vi "example_01_timescaledb.vi"() -> ()   [LabVIEW 2015, in "lv-timescaledb.lvlib"]
uses:
  lv-timescaledb.lvlib
  public/_controls/hypertable_options.ctl
  public/_controls/chunk.ctl
  public/_controls/time_type.ctl
  <vilib>/addons/database/Connection.llb/Conn ObjectReference.ctl
  <vilib>/addons/database/Connection.llb/DB Tools Open Connec (String).vi
  <vilib>/addons/database/NI_Database_API.lvlib
panel:
  out "connected?":bool
  in  "driver":string="PostgreSQL ANSI"
  in  "disconnect":bool
  in  "connect":bool
  in  "server":string="localhost"
  in  "password":string="timescaledb"
  in  "username":string="timescaledb"
  in  "chunk_name":string
  in  "hyper_table_name":string
  in  "tab_control":T1(tab)
  in  "hypertable_options":T2={"time_column"="time", "chunk_time_interval"=0.0} {"chunk_time_interval" format="%<%H:%M:%S>t"}
  in  "create_hypertable":bool
  in  "set_chunk_time_interval":bool
  in  "chunk_time_interval":dbl=86400.0 format="%<%H:%M:%S>t"
  in  "enable_compression":bool
  in  "segment_column":string="time"
  in  "disable_compression":bool
  in  "show_hyper_tables":bool
  out "hyper_tables":string[](array[string])
  in  "show_chunks":bool
  out "chunks_available []":T3[](array[typedef]) {"start" format="%^<%H:%M:%S%3u %m/%d/%y>T"; "end" format="%^<%H:%M:%S%3u %m/%d/%y>T"}
  out "decompressed_chunk":string
  out "compressed_chunk":string
  in  "decompress_chunk":bool
  in  "compress_chunk":bool
  in  "time_type":T4=enum."interval"
  in  "drop_chunks":bool
  out "chunks_dropped []":string[](array[string])
  in  "older_than_timestamp":dbl format="%^<%H:%M:%S%3u %m/%d/%y>T"
  in  "older_than_interval":dbl format="%<%H:%M:%S%4u>t"
  in  "newer_than_timestamp":dbl format="%^<%H:%M:%S%3u %m/%d/%y>T"
  in  "newer_than_interval":dbl format="%<%H:%M:%S%4u>t"
  in  "timezone":string
  in  "add_compression_policy":bool
  in  "add_retention_policy":bool
  in  "compression_interval":dbl=86400.0 format="%<%H:%M:%S%4u>t"
  in  "retention_interval":dbl=1.0 format="%<%H:%M:%S%4u>t"
  in  "remove_compression_policy":bool
  in  "remove_retention_policy":bool
  in  "stop":bool
  out "error":errorcluster
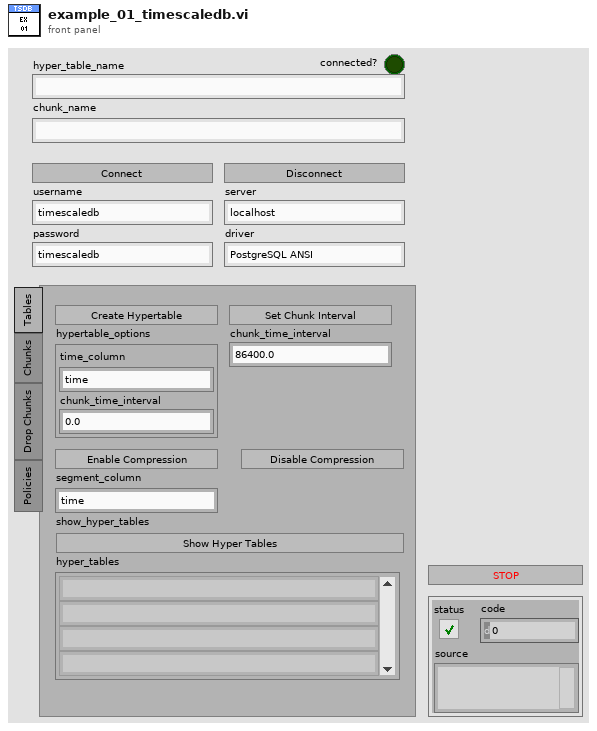
[diagram p1: front panel]
types:
  T1 = enum32{"Tables", "Chunks", "Drop Chunks", "Policies"}
  T2 = typedef "lv-timescaledb.lvlib/hypertable_options.ctl" = cluster{"time_column":string, "chunk_time_interval":dbl}
  T3 = typedef "lv-timescaledb.lvlib/chunk.ctl" = cluster{"name":string, "start":dbl, "end":dbl, "compressed":bool}
  T4 = typedef "lv-timescaledb.lvlib/time_type.ctl" = enum16{"<time_type>", "interval", "timestamp", "timestamp_with_timezone", "<null>"}
  T5 = typedef "NI_Database_API.lvlib/Conn ObjectReference.ctl" = refnum<k1>
  T6 = cluster{"timezone":string, "newer_than_interval":dbl}
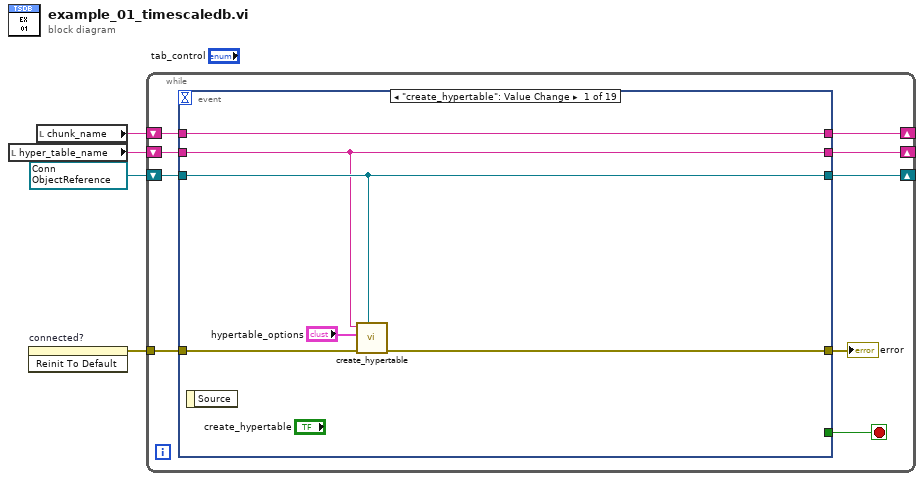
[diagram p0: block diagram]
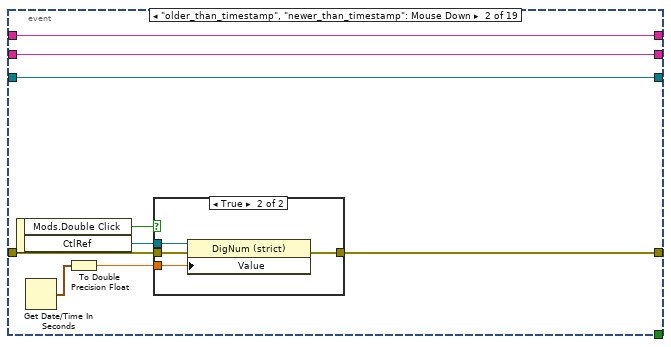
[diagram p2: hidden frame]
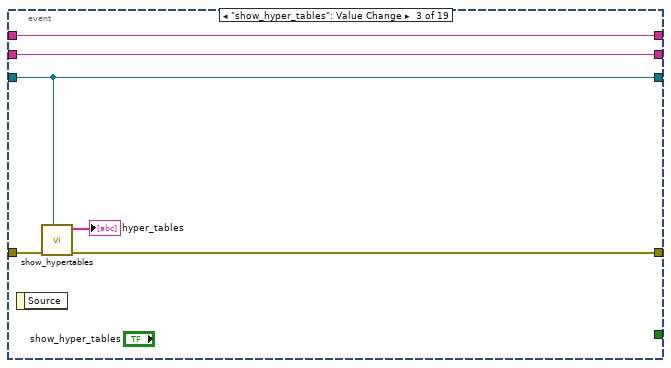
[diagram p4: hidden frame]
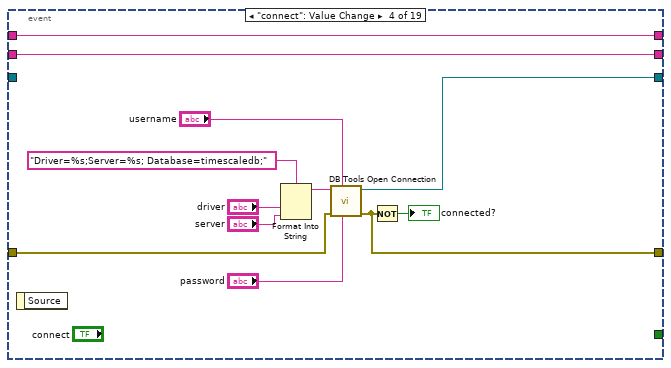
[diagram p5: hidden frame]
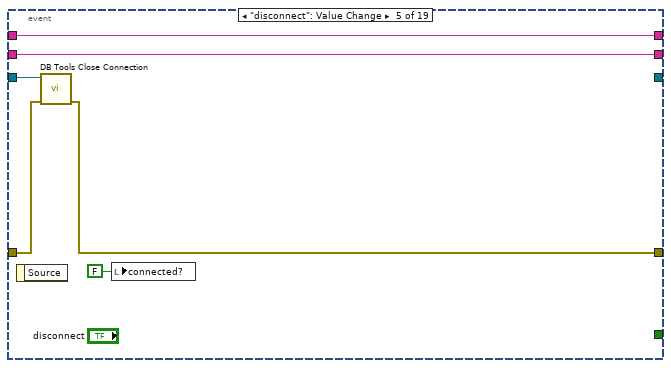
[diagram p6: hidden frame]
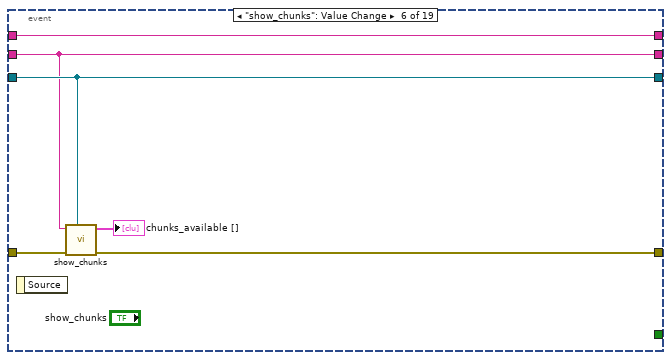
[diagram p7: hidden frame]
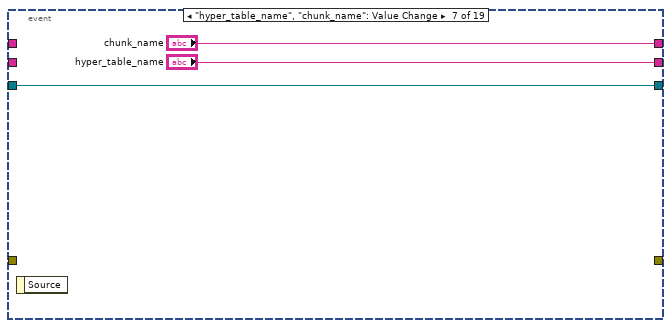
[diagram p8: hidden frame]
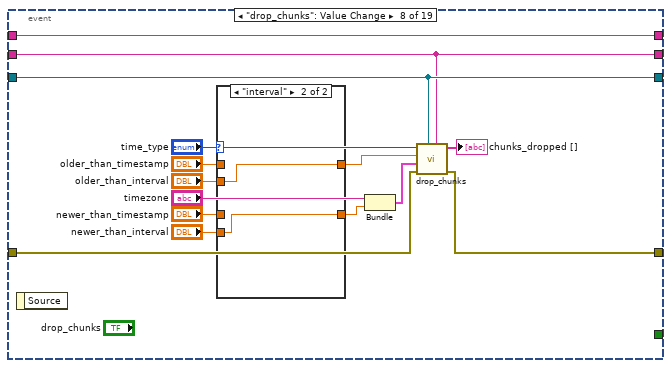
[diagram p9: hidden frame]
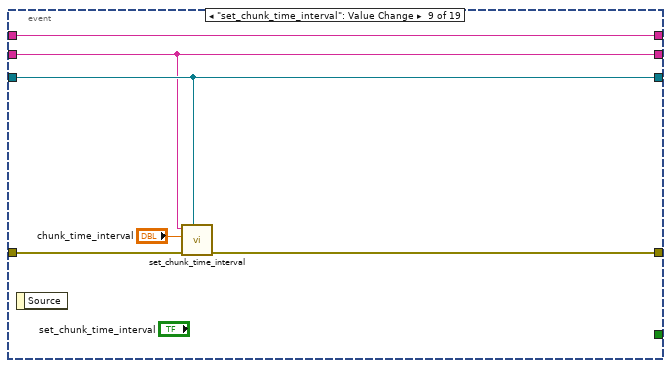
[diagram p11: hidden frame]
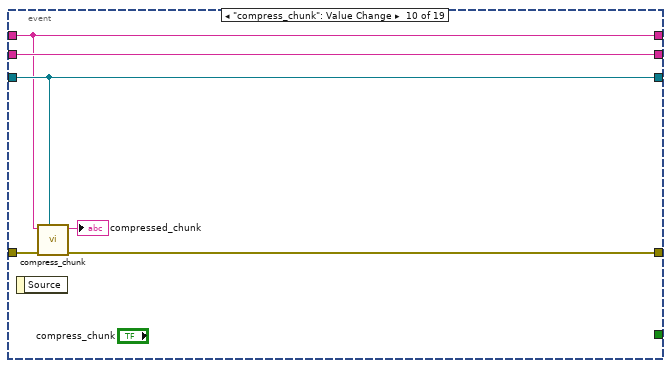
[diagram p12: hidden frame]
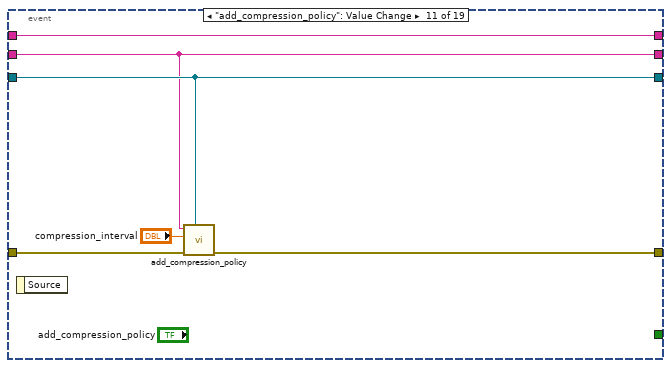
[diagram p13: hidden frame]
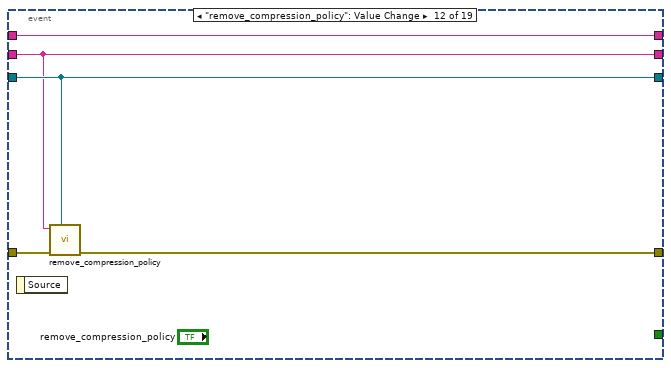
[diagram p14: hidden frame]
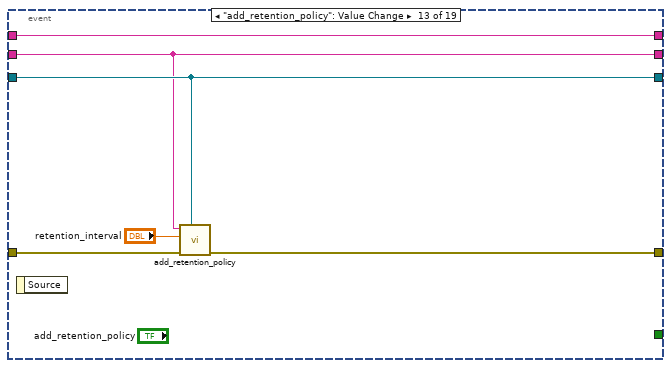
[diagram p15: hidden frame]
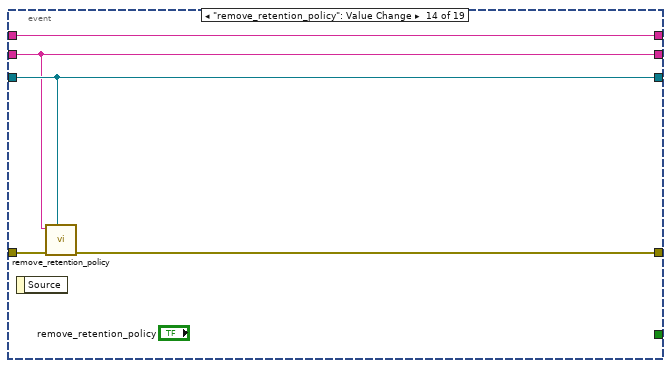
[diagram p16: hidden frame]
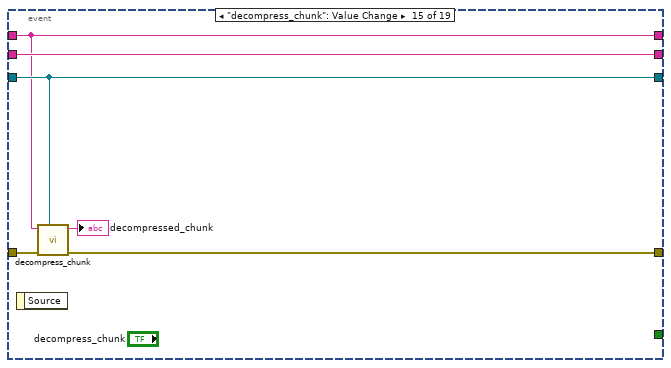
[diagram p17: hidden frame]
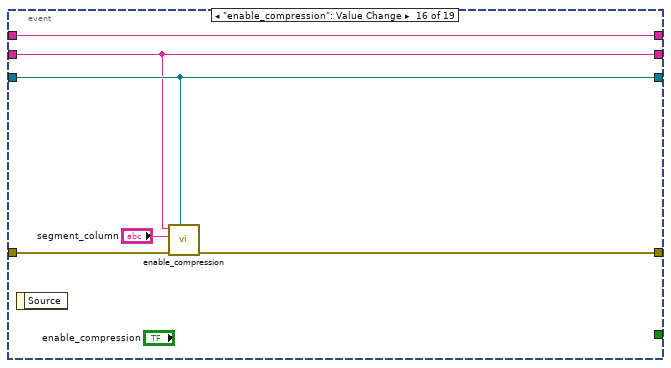
[diagram p18: hidden frame]
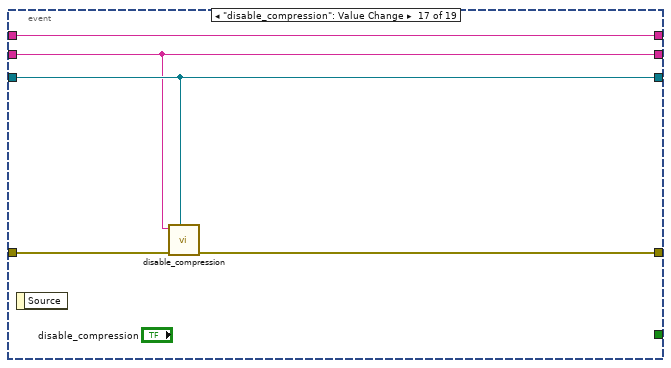
[diagram p19: hidden frame]
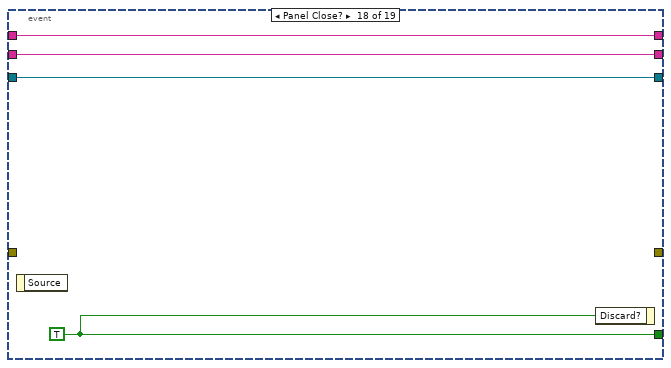
[diagram p20: hidden frame]
diagram:
  w3 = T5 refnum items=["Connection"] ("connection reference")
  n1 = local read "hyper_table_name"() -> (w4:string)
  n2 = invoke on="connected?" class="Bool (strict)" method="Reinit To Default"() -> (error out=w2:errorcluster)  [unwired: 3 in, 2 out]
  n3 = local read "chunk_name"() -> (w1:string)
  n4 = while {
    shift-right: [w10] -> _
    shift-left: w4 -> [w11]
    shift-right: [w9] -> _
    shift-left: w3 -> [w12]
    tunnel: w2 -> [w7]
    shift-right: [w5] -> _
    shift-left: w1 -> [w6]
    stop <- w13 stop-if-true
    n5 = event shown="[0] \"create_hypertable\": Value Change" {
      selector: _ -> [_ _ _ _ _ _ _ _ _ _ _ _ _ _ _ _ _ _ _]
      dyn-events: _ -> [_ _ _ _ _ _ _ _ _ _ _ _ _ _ _ _ _ _ _]
      timeout: _ -> [_ _ _ _ _ _ _ _ _ _ _ _ _ _ _ _ _ _ _]
      tunnel: [_ _ _ _ _ _ _ _ _ _ _ _ _ _ _ _ _ w140 TRUE] -> w13
      tunnel: [w19 w24 w37 w46 w55 w63 _ w81 w88 w94 w102 w105 w111 w117 w122 w129 w134 _ _] -> w8
      tunnel: w12 -> [w18 w27 w35 _ w56 w61 w65 w79 w91 w96 w101 w108 w114 w119 w124 w128 w133 w138 w142]
      tunnel: w11 -> [w16 w28 w39 w51 w57 w59 _ w73 w90 w97 w100 w107 w113 w116 w125 w127 w132 w139 w144]
      tunnel: [w16 w28 w39 w51 w57 w59 "hyper_table_name" w73 w90 w97 w100 w107 w113 w116 w125 w127 w132 w139 w144] -> w10
      tunnel: [w18 w27 w35 w47 _ w61 w65 w79 w91 w96 w101 w108 w114 w119 w124 w128 w133 w138 w142] -> w9
      tunnel: w7 -> [w17 w25 w38 w41 w53 w62 _ w80 w89 w95 w103 w106 w112 w118 w123 w130 w135 _ _]
      tunnel: w6 -> [w14 w20 w34 w40 w52 w58 _ w67 w86 w92 w98 w104 w109 w115 w120 w131 w136 w137 w141]
      tunnel: [w14 w20 w34 w40 w52 w58 "chunk_name" w67 w86 w92 w98 w104 w109 w115 w120 w131 w136 w137 w141] -> w5
      event "create_hypertable": Value Change {
        n6 = event-data() -> ()  [unwired: 1 in, 1 out]
        n7 = call "create_hypertable.vi"("connection_reference"=w18, "error in (no error)"=w17, "options"="hypertable_options", "table_name"=w16) -> ("error out"=w19:errorcluster)  [unwired: 6 in, 1 out]
      }
      event "older_than_timestamp", "newer_than_timestamp": Mouse Down {
        n8 = event-data() -> ("Mods.Double Click"=w21:bool, "CtlRef"=w26:refnum<vi>)  [unwired: 1 in]
        n9 = Get Date/Time In Seconds() -> (seconds since 1Jan1904=w23:timestamp)
        n10 = To Double Precision Float(number=w23) -> (double precision float=w22:dbl)
        n11 = case shown="True" w21 {
          tunnel: w26 -> [_ w33]
          tunnel: w25 -> [w29 w32]
          tunnel: [w29 w31] -> w24
          tunnel: w22 -> [_ w30]
          frame False {
          }
          frame True {
            n12 = property class="DigNum (strict)"(reference=w33, error in=w32, "Value"=w30) -> (error out=w31:errorcluster)  [unwired: 1 out]
          }
        }
      }
      event "show_hyper_tables": Value Change {
        n13 = event-data() -> ()  [unwired: 1 in, 1 out]
        n14 = call "show_hypertables.vi"("connection_reference"=w35, "error in (no error)"=w38) -> ("error out"=w37:errorcluster, "hyper_table_names []"=→"hyper_tables":string[])  [unwired: 8 in]
      }
      event "connect": Value Change {
        n15 = event-data() -> ()  [unwired: 1 in, 1 out]
        n16 = Format Into String(format string="Driver=%s;Server=%s; Database=timescaledb;", "driver", "server") -> (resulting string=w50:string)  [unwired: 2 in, 1 out]
        n17 = call-poly <vilib>:"DB Tools Open Connection.vi"("password"="password", "userID"="username", "error in (no error)"=w41, "connection information"=w50) -> ("error out"=w46:errorcluster, "connection reference"=w47:T5)  [unwired: 4 in]
        n18 = Not(x=w46) -> (.not. x?=→"connected?":bool)
      }
      event "disconnect": Value Change {
        n19 = event-data() -> ()  [unwired: 1 in, 1 out]
        n20 = call <vilib>:"DB Tools Close Connection.vi"("error in (no error)"=w53, "connection reference"=w56) -> ("error out"=w55:errorcluster)  [unwired: 5 in]
        n21 = local write "connected?"(FALSE ("connected?")) -> ()
      }
      event "show_chunks": Value Change {
        n22 = event-data() -> ()  [unwired: 1 in, 1 out]
        n23 = call "show_chunks.vi"("connection_reference"=w61, "error in (no error)"=w62, "hyper_table_name"=w59) -> ("error out"=w63:errorcluster, "chunk []"=→"chunks_available []":T3[])  [unwired: 7 in]
      }
      event "hyper_table_name", "chunk_name": Value Change {
        n24 = event-data() -> ()  [unwired: 1 in, 1 out]
      }
      event "drop_chunks": Value Change {
        n25 = event-data() -> ()  [unwired: 1 in, 1 out]
        n26 = case shown="\"interval\"" "time_type" {
          tunnel: "older_than_timestamp" -> [w83 _]
          tunnel: "older_than_interval" -> [_ w85]
          tunnel: [w83 w85] -> w75
          tunnel: "newer_than_timestamp" -> [w82 _]
          tunnel: "newer_than_interval" -> [_ w84]
          tunnel: [w82 w84] -> w69
          frame Default {
          }
          frame "interval" {
          }
        }
        n27 = Bundle("timezone"="timezone", "newer_than_interval"=w69) -> (w68:T6)  [unwired: 1 in]
        n28 = call "drop_chunks.vi"("hyper_table_name"=w73, "connection_reference"=w79, "error in (no error)"=w80, "chunk_options"=w68, "older_than"=w75, "time_type"="time_type") -> ("error out"=w81:errorcluster, "chunks_dropped []"=→"chunks_dropped []":string[])  [unwired: 4 in]
      }
      event "set_chunk_time_interval": Value Change {
        n29 = event-data() -> ()  [unwired: 1 in, 1 out]
        n30 = call "set_chunk_time_interval.vi"("connection_reference"=w91, "error in (no error)"=w89, "chunk_time_interval"="chunk_time_interval", "hyper_table_name"=w90) -> ("error out"=w88:errorcluster)  [unwired: 7 in]
      }
      event "compress_chunk": Value Change {
        n31 = event-data() -> ()  [unwired: 1 in, 1 out]
        n32 = call "compress_chunk.vi"("connection_reference"=w96, "error in (no error)"=w95, "chunk_name"=w92) -> ("error out"=w94:errorcluster, "compressed_chunk"=→"compressed_chunk":string)  [unwired: 7 in]
      }
      event "add_compression_policy": Value Change {
        n33 = event-data() -> ()  [unwired: 1 in, 1 out]
        n34 = call "add_compression_policy.vi"("connection_reference"=w101, "error in (no error)"=w103, "compression_interval"="compression_interval", "hyper_table_name"=w100) -> ("error out"=w102:errorcluster)  [unwired: 7 in]
      }
      event "remove_compression_policy": Value Change {
        n35 = event-data() -> ()  [unwired: 1 in, 1 out]
        n36 = call "remove_compression_policy.vi"("connection_reference"=w108, "error in (no error)"=w106, "hyper_table_name"=w107) -> ("error out"=w105:errorcluster)  [unwired: 8 in]
      }
      event "add_retention_policy": Value Change {
        n37 = event-data() -> ()  [unwired: 1 in, 1 out]
        n38 = call "add_retention_policy.vi"("connection_reference"=w114, "error in (no error)"=w112, "retention_interval"="retention_interval", "hyper_table_name"=w113) -> ("error out"=w111:errorcluster)  [unwired: 7 in]
      }
      event "remove_retention_policy": Value Change {
        n39 = event-data() -> ()  [unwired: 1 in, 1 out]
        n40 = call "remove_retention_policy.vi"("connection_reference"=w119, "error in (no error)"=w118, "hyper_table_name"=w116) -> ("error out"=w117:errorcluster)  [unwired: 8 in]
      }
      event "decompress_chunk": Value Change {
        n41 = event-data() -> ()  [unwired: 1 in, 1 out]
        n42 = call "decompress_chunk.vi"("connection_reference"=w124, "error in (no error)"=w123, "chunk_name"=w120) -> ("error out"=w122:errorcluster, "decompressed_chunk"=→"decompressed_chunk":string)  [unwired: 7 in]
      }
      event "enable_compression": Value Change {
        n43 = event-data() -> ()  [unwired: 1 in, 1 out]
        n44 = call "enable_compression.vi"("connection_reference"=w128, "error in (no error)"=w130, "segment_column"="segment_column", "hyper_table_name"=w127) -> ("error out"=w129:errorcluster)  [unwired: 7 in]
      }
      event "disable_compression": Value Change {
        n45 = event-data() -> ()  [unwired: 1 in, 1 out]
        n46 = call "disable_compression.vi"("connection_reference"=w133, "error in (no error)"=w135, "hyper_table_name"=w132) -> ("error out"=w134:errorcluster)  [unwired: 8 in]
      }
      event Panel Close? {
        w140 = TRUE
        n47 = event-data() -> ()  [unwired: 1 in, 1 out]
        n48 = event-data("Discard?"=w140) -> ()  [unwired: 1 in, 1 out]
      }
      event "stop": Value Change {
        n49 = event-data() -> ()  [unwired: 1 in, 1 out]
      }
    }
    "error" <- w8
  }
